vi "ConvertTextBasedCodeToLabVIEW_GetDataTypeNames.vi"(9 "EnumsOusideClass":T11[](array[typedef]), 10 "StructsOusideClass":T12[](array[typedef]), 11 "Classes":T1[](array[typedef])) -> (2 "DataType:Name":string[](array[string]), 3 "DataType:Type":T6[](array[typedef]))   [LabVIEW 2020]
uses:
  <resource>/Framework/Providers/Open_GDS/ClassProviders/Common/CommonVIs/CommonVIs_EnumType.ctl
  <resource>/Framework/Providers/Open_GDS/ClassProviders/Common/String/GDSString_AccessScopeModifierType.ctl
  <resource>/Framework/Providers/Open_GDS/ClassProviders/Common/String/GDSString_ModifierType.ctl
  <resource>/Framework/Providers/Open_GDS/ClassProviders/Common/CommonVIs/CommonVIs_StructType.ctl
  <resource>/Framework/Providers/Open_GDS/ClassProviders/Common/CommonVIs/CommonVIs_AttributeType.ctl
  <resource>/Framework/Providers/Open_GDS/ClassProviders/Common/CommonVIs/CommonVIs_AttributeDataType.ctl
  <resource>/Framework/Providers/Open_GDS/ClassProviders/Common/String/GDSString_ClassDescriptionType.ctl
  <resource>/Framework/Providers/Open_GDS/ClassProviders/Common/String/GDSString_MethodDescriptionType.ctl
  <resource>/Framework/Providers/Open_GDS/ClassProviders/Common/CommonVIs/CommonVIs_PropertyType.ctl
  <resource>/Framework/Providers/Open_GDS/ClassProviders/Common/String/GDSString_ClassParentType.ctl
  <resource>/Framework/Providers/Open_GDS/ClassProviders/Common/String/GDSString_ClassType.ctl
  <resource>/Framework/Providers/Open_GDS/ClassProviders/Common/String/GDSString_ClassOwnerType.ctl
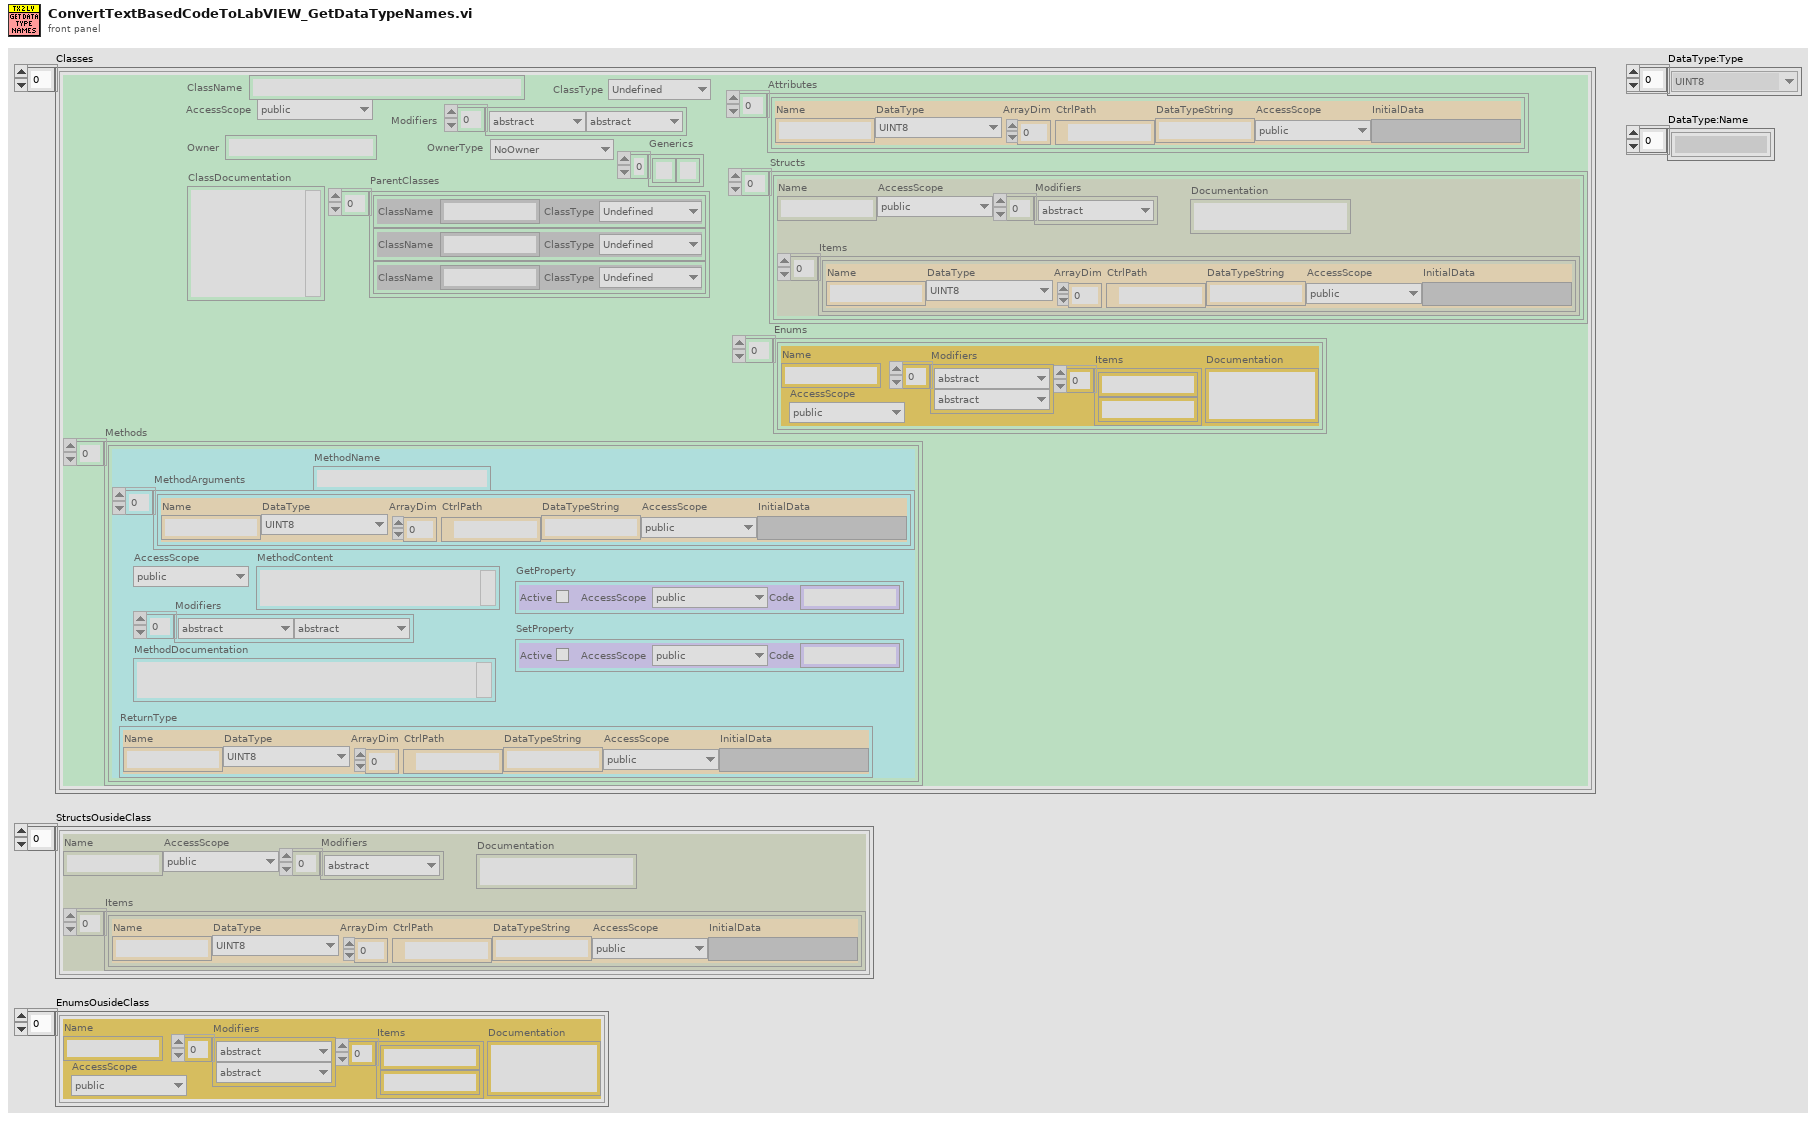
[diagram p1: front panel]
types:
  T1 = typedef "GDSString_ClassDescriptionType.ctl" = cluster{"ClassName":string, "AccessScope":T2, "Modifiers":T3[], "ClassDocumentation":string, "Methods":T4[], "ParentClasses":T8[], "ClassType":T9, "Owner":string, "OwnerType":T10, "Generics":string[], "Attributes":T5[], "Enums":T11[], "Structs":T12[]}
  T2 = typedef "GDSString_AccessScopeModifierType.ctl" = enum16{"public", "private", "protected", "internal"}
  T3 = typedef "GDSString_ModifierType.ctl" = enum16{"abstract", "static", "final", "synchronized", "strictfp", "async", "const", "event", "extern", "new", "native ", "override", "partial", "readonly", "sealed", "unsafe", "virtual", "volatile"}
  T4 = typedef "GDSString_MethodDescriptionType.ctl" = cluster{"ReturnType":T5, "MethodName":string, "AccessScope":T2, "Modifiers":T3[], "MethodDocumentation":string, "MethodContent":string, "MethodArguments":T5[], "GetProperty":T7, "SetProperty":T7}
  T5 = typedef "CommonVIs_AttributeType.ctl" = cluster{"Name":string, "DataType":T6, "ArrayDim":i32, "CtrlPath":path, "DataTypeString":string, "AccessScope":T2, "InitialData":variant}
  T6 = typedef "CommonVIs_AttributeDataType.ctl" = enum16{"UINT8", "INT8", "UINT16", "INT16", "UINT32", "INT32", "UINT64", "INT64", "SGL", "DBL", "EXT", "CSG", "CDB", "CXT", "TimeStamp", "STRING", "PATH", "BOOL", "ENUM", "RefNum", "VIRefNum", "LabVIEW Class", "Cluster", "Variant", "TypeDef", "Waveform", "LabVIEW Object", "Other", "void", "Set", "Map"}
  T7 = typedef "CommonVIs_PropertyType.ctl" = cluster{"Active":bool, "AccessScope":T2, "Code":string}
  T8 = typedef "GDSString_ClassParentType.ctl" = cluster{"ClassName":string, "ClassType":T9}
  T9 = typedef "GDSString_ClassType.ctl" = enum16{"Undefined", "Class", "Interface"}
  T10 = typedef "GDSString_ClassOwnerType.ctl" = enum16{"NoOwner", "Class", "Package/NameSpace"}
  T11 = typedef "CommonVIs_EnumType.ctl" = cluster{"Name":string, "AccessScope":T2, "Modifiers":T3[], "Items":string[], "Documentation":string}
  T12 = typedef "CommonVIs_StructType.ctl" = cluster{"Name":string, "AccessScope":T2, "Modifiers":T3[], "Items":T5[], "Documentation":string}
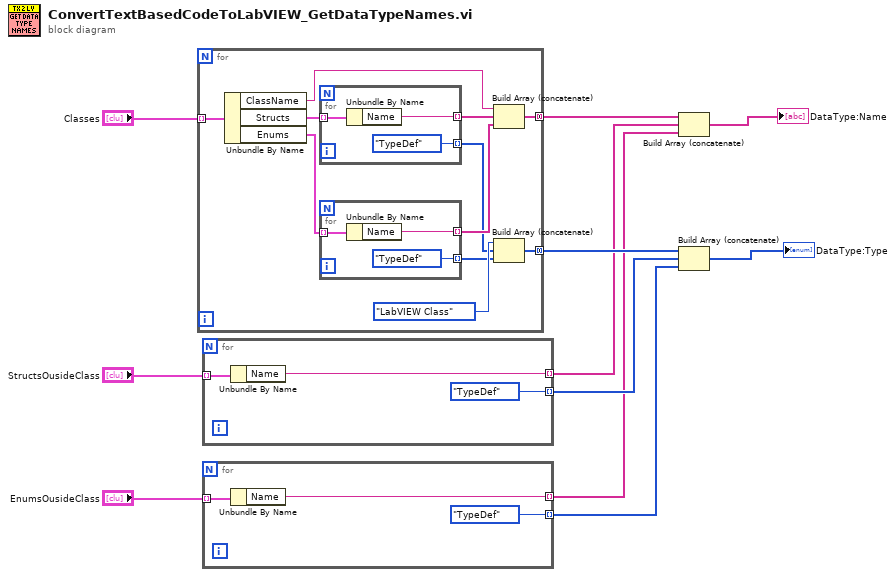
[diagram p0: block diagram]
diagram:
  n1 = for {
    tunnel: "Classes" -> [w22] mode=indexing
    tunnel: [w18] -> w10 mode=concatenating
    tunnel: [w12] -> w11 mode=concatenating
    n2 = Unbundle By Name(w22) -> ("ClassName"=w21:string, "Structs"=w20:T12[], "Enums"=w19:T11[])
    n3 = for {
      tunnel: w20 -> [w28] mode=indexing
      tunnel: [w27] -> w17 mode=indexing
      tunnel: [CommonVIs_AttributeDataType."TypeDef" ("DataType")] -> w14 mode=indexing
      n4 = Unbundle By Name(w28) -> ("Name"=w27:string)
    }
    n5 = for {
      tunnel: w19 -> [w25] mode=indexing
      tunnel: [w24] -> w16 mode=indexing
      tunnel: [CommonVIs_AttributeDataType."TypeDef" ("DataType")] -> w13 mode=indexing
      n6 = Unbundle By Name(w25) -> ("Name"=w24:string)
    }
    n7 = Build Array (concatenate)(w21, w17, w16) -> (w18:string[])
    n8 = Build Array (concatenate)(CommonVIs_AttributeDataType."LabVIEW Class" ("DataType"), w14, w13) -> (w12:T6[])
  }
  n9 = for {
    tunnel: "StructsOusideClass" -> [w31] mode=indexing
    tunnel: [w30] -> w5 mode=indexing
    tunnel: [CommonVIs_AttributeDataType."TypeDef" ("DataType")] -> w4 mode=indexing
    n10 = Unbundle By Name(w31) -> ("Name"=w30:string)
  }
  n11 = for {
    tunnel: "EnumsOusideClass" -> [w34] mode=indexing
    tunnel: [w33] -> w2 mode=indexing
    tunnel: [CommonVIs_AttributeDataType."TypeDef" ("DataType")] -> w1 mode=indexing
    n12 = Unbundle By Name(w34) -> ("Name"=w33:string)
  }
  n13 = Build Array (concatenate)(w10, w5, w2) -> (→"DataType:Name":string[])
  n14 = Build Array (concatenate)(w11, w4, w1) -> (→"DataType:Type":T6[])
